vi "acquisition test fixed exposure 4.vi"() -> ()   [LabVIEW 2023]
uses:
  <vilib>/vision/driver/IMAQdx.llb/IMAQdx Attribute Type.ctl
  <vilib>/userDefined/High Color/IMAQdx.ctl
  <vilib>/vision/driver/IMAQdx.llb/IMAQdx Acquisition Mode.ctl
  Program Files/NI/LVAddons/niimaqdx/1/examples/Vision Acquisition/NI-IMAQdx/Stream to Disk/SubVIs/TDMS Write Settings.ctl
  <vilib>/vision/Image Controls.llb/IMAQ Image.ctl
  <vilib>/vision/driver/IMAQdx.llb/IMAQdx Buffer Number Mode.ctl
  <vilib>/DAQmx/read.llb/DAQmx Read (Analog 1D Wfm NChan NSamp).vi
  <extravilib>/ChannelInstances/Tag-bool/Read With Abort.vi
  <vilib>/Utility/High Resolution Relative Seconds.vi
  <extravilib>/ChannelInstances/Tag-bool/Write With Abort.vi
  <vilib>/DAQmx/create/channels.llb/DAQmx Create Channel (AI-Voltage-Basic).vi
  <vilib>/DAQmx/configure/timing.llb/DAQmx Timing (Sample Clock).vi
  Program Files/NI/LVAddons/niimaqdx/1/examples/Vision Acquisition/NI-IMAQdx/Stream to Disk/SubVIs/TDMS File Initialization (Write).vi
  <extravilib>/ChannelInstances/Tag-bool/Instantiate.vi
  <extravilib>/ChannelInstances/Tag-bool/EndpointRead.vi
  <vilib>/vision/EDVR.llb/IMAQ ImageToEDVR.vi
  <vilib>/vision/EDVR.llb/IMAQ ImageToEDVR 1D U8.vi
  <vilib>/vision/EDVR.llb/IMAQ ImageToEDVR 1D I16.vi
  <vilib>/vision/EDVR.llb/IMAQ ImageToEDVR 1D U32.vi
  <vilib>/vision/EDVR.llb/IMAQ ImageToEDVR 1D U16.vi
  <extravilib>/ChannelInstances/Tag-bool/Endpoint.vi
  <vilib>/DAQmx/miscellaneous.llb/DAQmx Fill In Error Info.vi
  <extravilib>/ChannelInstances/Tag-bool.lvlib
  <vilib>/vision/driver/NI_Vision_Acquisition_Software.lvlib
  <resource>/objmgr/imaqdx.rc
panel:
  out "error out":errorcluster
  in  "Image Type":u16(ring) items=["Grayscale (U8)"=0, "Grayscale (I16)"=1, "Grayscale (U16)"=7, "RGB Color (U32)"=4]
  out "Image 2":T1(plugin-control)
  in  "Buffer Images":i32=30
  out "Optimizations":T2
  in  "Images per TDMS":i64=10000
  out "Images Behind 2":u32
  out "Write Speed":dbl(graph) caption="Image File Write Speed"
  out "Images Acquired Per Second":dbl
  out "Images Saved Per Second":dbl
  out "Destination Folder":path
  out "Maximum FrameRate":dbl
  out "Attribute Information":T4
  out "Sensor Readout Time":dbl
  out "Waveform Chart":waveform(dbl)[](graph)
  in  "stop collection":bool
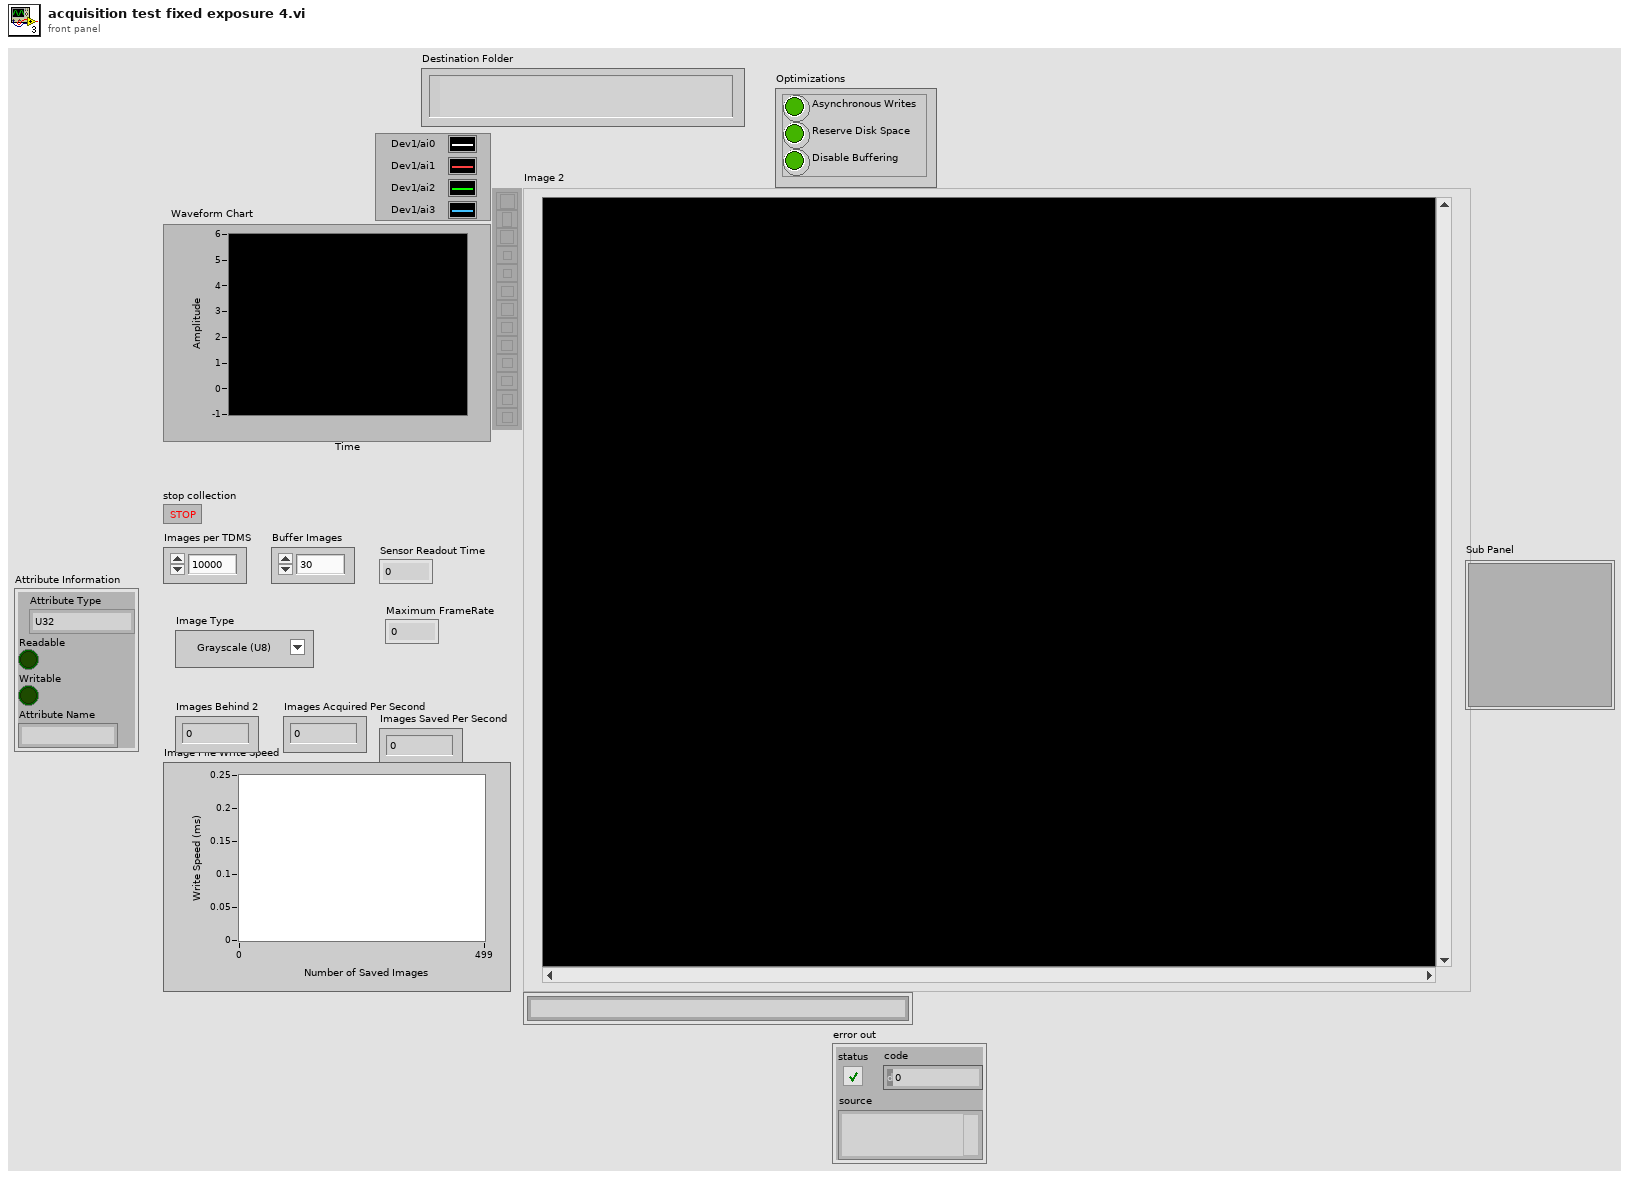
[diagram p1: front panel]
types:
  T1 = typedef "IMAQ Image.ctl" = refnum<image>
  T2 = cluster{"Asynchronous Writes":bool, "Reserve Disk Space":bool, "Disable Buffering":bool}
  T3 = typedef "NI_Vision_Acquisition_Software.lvlib/IMAQdx Attribute Type.ctl" = enum32{"U32", "I64", "DBL", "String", "Enum", "Bool", "Command"}
  T4 = cluster{"Attribute Type":T3, "Readable":bool, "Writable":bool, "Attribute Name":string}
  T5 = typedef "TDMS Write Settings.ctl" = cluster{"Asynchronous":bool, "Disable Buffering if Supported":bool, "Reserved Images":i64, "Fail if Reservation Fails":bool}
  T6 = typedef "NI_Vision_Acquisition_Software.lvlib/IMAQdx Acquisition Mode.ctl" = enum32{"One Shot", "Continuous"}
  T7 = enum16{"Exposure End", "Exposure Center", "Exposure Start", "Start", "NoSync"}
  T8 = typedef "IMAQdx.ctl" = refnum<k21>
  T9 = cluster{"Attribute Type":T3, "Readable":bool, "Writable":bool, "Attribute Name":string}[]
  T10 = typedef "Image Type" = u32
  T11 = cluster{"Image Type":T10, "Async File Format":bool}
  T12 = cluster{"Asynchronous Write":bool, "Reserve Disk Space":bool, "Disable Buffering":bool}
  T13 = typedef "Tag-bool.lvlib/))Channel.ctl" = refnum<queue>
  T14 = typedef "NI_Vision_Acquisition_Software.lvlib/IMAQdx Buffer Number Mode.ctl" = enum32{"Next", "Last", "Buffer Number", "Every", "Last New"}
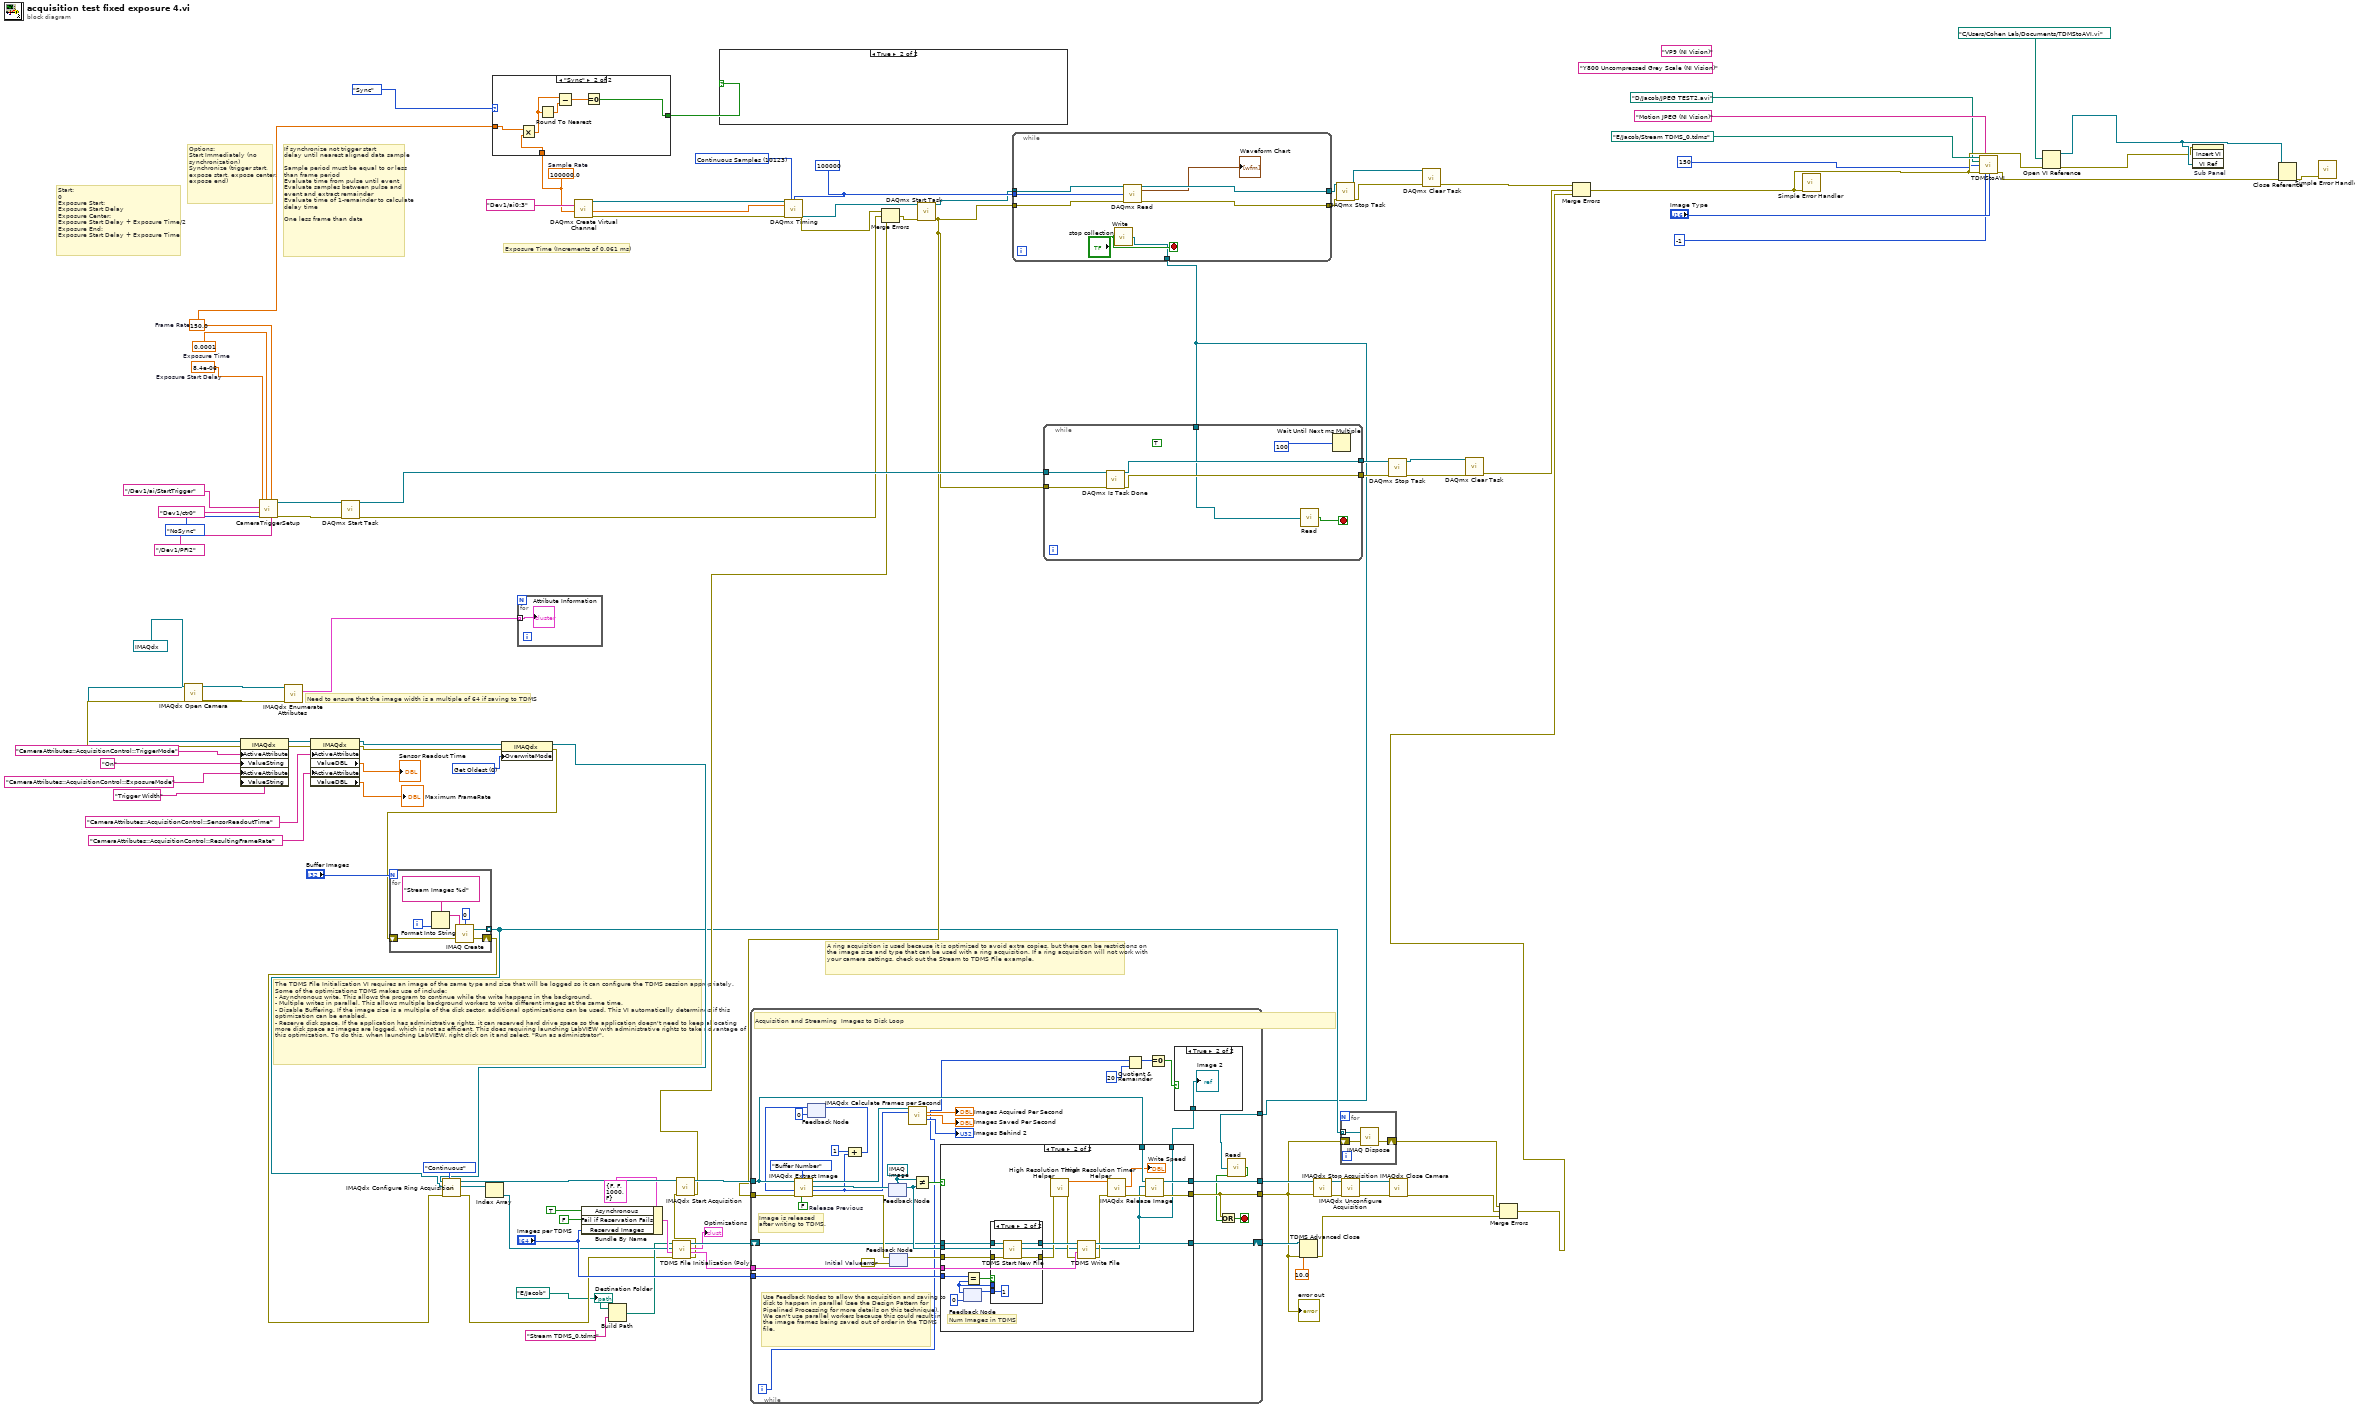
[diagram p0: block diagram]
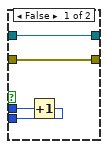
[diagram p4: hidden frame]
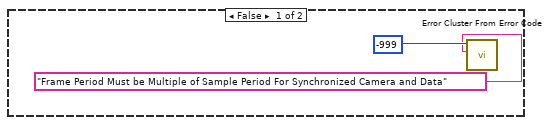
[diagram p5: hidden frame]
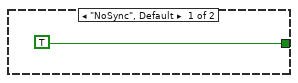
[diagram p6: hidden frame]
diagram:
  w6 = path "E:/Jacob" ("Destination Folder")
  (unwired) "Y800 Uncompressed Grey Scale (NI Vision)" ("Codec")
  (unwired) "VP9 (NI Vision)" ("Codec")
  w33 = u32 0 items=["Get Oldest"=0, "Fail"=2, "Get Newest"=3] ("OverwriteMode")
  w71 = 8.4e-06  # Exposure Start Delay
  w67 = 150.0  # Frame Rate
  w70 = 0.0001  # Exposure Time
  w98 = 10123 items=["Finite Samples"=10178, "Continuous Samples"=10123, "Hardware Timed Single Point"=12522] ("sample mode")
  w99 = 100000 ("number of samples per channel")
  w68 = 100000.0  # Sample Rate
  # "Need to ensure that the image width is a multiple of 64 if saving to TDMS"
  # "The TDMS File Initialization VI requires an image of the same type and size that will be logged so it can configure the TDMS session appropriately. Some of the optimizations TDMS makes use of include:\n- Asynchronous write. This allows the program to continue while the write happens in the background.\n- Multiple writes in parallel. This allows multiple background workers to write different images at the same time.\n- Disable Buffering. If the image size is a multiple of the disk sector, additional optimizations can be used. This VI automatically determines if this optimization can be enabled.\n- Reserve disk space. If the application has administrative rights, it can reserved hard drive space so the application doesn't need to keep allocating more disk space as images are logged, which is not as efficient. This does requiring launching LabVIEW with administrative rights to take advantage of this optimization. To do this, when launching LabVIEW, right click on it and select, \"Run as administrator\"."
  # "A ring acquisition is used because it is optimized to avoid extra copies, but there can be restrictions on the image size and type that can be used with a ring acquisition. If a ring acquisition will not work with your camera settings, check out the Stream to TDMS File example."
  # "Start:\n0\nExposure Start:\nExposure Start Delay\nExposure Center:\nExposure Start Delay + Exposure Time/2\nExposure End:\nExposure Start Delay + Exposure Time"
  # "If synchronize not trigger start\ndelay until nearest aligned data sample\n\nSample period must be equal to or less than frame period\nEvaluate time from pulse until event\nEvaluate samples between pulse and event and extract remainder\nEvaluate time of 1-remainder to calculate delay time\n\nOne less frame than data"
  # "Options:\nStart Immediately (no synchronization)\nSynchronize (trigger start, expose start, expose center, expose end)"
  # "Exposure Time (Increments of 0.061 ms)"
  n1 = call <vilib>:"IMAQdx Open Camera.vi"("Session In"=T8 "cam0") -> ("error out"=w89:errorcluster, "Session Out"=w94:T8)  [unwired: 9 in]
  n2 = call "CameraTriggerSetup.vi"("Camera\nTrigger\nOutput"=tag "/Dev1/PFI2" ("CO.Pulse.Term"), "Frame Rate"=w67, "Sync Type"=T7."NoSync", "Exposure Time"=w70, "Camera\nClock\nCounter"=tag "Dev1/ctr0" ("counter"), "Start Trigger Source"=tag "/Dev1/ai/StartTrigger" ("source"), "Exposure Start Delay"=w71) -> ("error out"=w64:errorcluster, "Refnum out"=w65:refnum<k21>)  [unwired: 3 in]
  n3 = call <vilib>:"IMAQdx Enumerate Attributes.vi"("error in"=w89, "Session In"=w94) -> ("error out"=w93:errorcluster, "Attribute Information Array"=w84:T9, "Session Out"=w92:T8)  [unwired: 7 in]
  n4 = property class="IMAQdx"(reference=w92, error in=w93, "ActiveAttribute"="CameraAttributes::AcquisitionControl::TriggerMode", "ValueString"="On", "ActiveAttribute"="CameraAttributes::AcquisitionControl::ExposureMode", "ValueString"="Trigger Width") -> (reference out=w86:T8, error out=w85:errorcluster)
  n5 = property class="IMAQdx"(reference=w86, error in=w85, "ActiveAttribute"="CameraAttributes::AcquisitionControl::SensorReadoutTime", "ActiveAttribute"="CameraAttributes::AcquisitionControl::ResultingFrameRate") -> (reference out=w32:T8, error out=w31:errorcluster, "ValueDBL"=→"Sensor Readout Time":dbl, "ValueDBL"=→"Maximum FrameRate":dbl)
  n6 = call <vilib>:"DAQmx Start Task.vi"("task/channels in"=w65, "error in"=w64) -> ("task out"=w63:refnum<k21>, "error out"=w58:errorcluster)  [unwired: 12 in]
  n7 = case shown="\"Sync\"" enum16{"NoSync", "Sync"}."Sync" {
    tunnel: [TRUE w104] -> w66
    tunnel: w67 -> [_ w109]
    tunnel: w68 -> [_ w108]
    frame "NoSync", Default {
    }
    frame "Sync" {
      n8 = Multiply(x=w109, y=w108) -> (x*y=w105:dbl)
      n9 = Round To Nearest(number=w105) -> (nearest integer value=w107:dbl)
      n10 = Subtract(x=w105, y=w107) -> (x-y=w106:dbl)
      n11 = Equal To 0?(x=w106) -> (x = 0?=w104:bool)
    }
  }
  n12 = property class="IMAQdx"(reference=w32, error in=w31, "OverwriteMode"=w33) -> (reference out=w25:T8, error out=w29:errorcluster)
  n13 = for {
    N: "Buffer Images" -> [_]
    tunnel: [w115] -> w23 mode=indexing
    shift-right: [w114] -> w24
    shift-left: w29 -> [w116]
    i -> [w113]
    n14 = Format Into String(format string="Stream Images %d" ("Image Name"), w113) -> (resulting string=w112:string)  [unwired: 2 in, 1 out]
    n15 = call "IMAQ Create"("Border Size"=0, "Image Name"=w112, "error in (no error)"=w116) -> ("New Image"=w115:T1, "error out"=w114:errorcluster)  [unwired: 1 in, 1 out]
  }
  n16 = call <vilib>:"IMAQdx Configure Ring Acquisition.vi"("Mode"=IMAQdx_Acquisition_Mode."Continuous" ("Continuous?"), "error in"=w24, "Images"=w23, "Session In"=w25) -> ("error out"=w7:errorcluster, "Images Out"=w36:T1[], "Session Out"=w49:T8)  [unwired: 5 in]
  n17 = Index Array(array=w36) -> (element=w35:T1)  [unwired: 1 in]
  n18 = for {
    tunnel: w84 -> [w117] mode=indexing
    "Attribute Information" <- w117
  }
  n19 = call-poly <vilib>:"DAQmx Create Virtual Channel.vi"("physical channels"=tag "Dev1/ai0:3") -> ("task out"=w102:refnum<k21>, "error out"=w101:errorcluster)  [unwired: 13 in]
  n20 = Bundle By Name(cluster=T5 {"Asynchronous"=FALSE, "Disable Buffering if Supported"=FALSE, "Reserved Images"=1000, "Fail if Reservation Fails"=FALSE} ("Write Settings"), "Asynchronous"=TRUE, "Fail if Reservation Fails"=FALSE, "Reserved Images"="Images per TDMS") -> (w39:T5)
  n21 = Build Path(base path=w6, name or relative path="Stream TDMS_0.tdms") -> (appended path=w20:path)
  n22 = call-poly "TDMS File Initialization (Poly).vi"("error in (no error)"=w7, "Write Settings"=w39, "Image In"=w35, "File Path"=w20) -> ("error out"=w34:errorcluster, "Write Settings Out"=w42:T11, "Optimizations Configured"=→"Optimizations":T12, "TDMS Refnum Out"=w44:refnum<k34>)  [unwired: 4 in]
  n23 = call <vilib>:"IMAQdx Start Acquisition.vi"("error in"=w34, "Session In"=w49) -> ("error out"=w27:errorcluster, "Session Out"=w46:T8)  [unwired: 8 out]
  n24 = case shown="True" w66 {
    frame False {
      n25 = call <vilib>:"Error Cluster From Error Code.vi"("error message (\"\")"="Frame Period Must be Multiple of Sample Period For Synchronized Camera and Data" ("source"), "error code (0)"=-999 ("code")) -> ()  [unwired: 7 in, 1 out]
    }
    frame True {
    }
  }
  n26 = call-poly <vilib>:"DAQmx Timing.vi"("task/channels in"=w102, "sample mode"=w98, "samples per channel"=w99, "rate"=w68, "error in"=w101) -> ("task out"=w62:refnum<k21>, "error out"=w60:errorcluster)  [unwired: 9 in]
  n27 = Merge Errors(w60, w58, w27) -> (w59:errorcluster)
  n28 = call <vilib>:"DAQmx Start Task.vi"("task/channels in"=w62, "error in"=w59) -> ("task out"=w61:refnum<k21>, "error out"=w26:errorcluster)  [unwired: 12 in]
  n29 = while {
    tunnel: [w127] -> w82
    tunnel: [w126] -> w81
    tunnel: w61 -> [w125]
    tunnel: w26 -> [w124]
    tunnel: w99 -> [w123]
    tunnel: [w120] -> w22
    stop <- "stop collection" stop-if-true
    n30 = call <extravilib>:"Write.vi"("element"="stop collection") -> ("channel"=w120:T13)  [unwired: 1 out]
    n31 = call-poly <vilib>:"DAQmx Read.vi"("task/channels in"=w125, "number of samples per channel"=w123, "error in"=w124) -> ("task out"=w127:refnum<k21>, "data"=→"Waveform Chart":waveform(dbl)[], "error out"=w126:errorcluster)  [unwired: 10 in]
  }
  n32 = while {
    tunnel: w26 -> [w161]
    tunnel: w46 -> [w158]
    tunnel: [w159] -> w47
    tunnel: [w147] -> w12
    shift-right: [w160] -> w41
    shift-left: w44 -> [w144]
    tunnel: "Images per TDMS" -> [w143]
    tunnel: w42 -> [w146]
    tunnel: w22 -> [w129]
    i -> [w131]
    stop <- w149 stop-if-true
    w135 = errorcluster {"status"=FALSE, "code"=0, "source"=""}  # Initial Value
    w156 = FALSE  # Release Previous
    w152 = T1 refnum ("Image Out")
    # "Use Feedback Nodes to allow the acquisition and saving to disk to happen in parallel (see the Design Pattern for Pipelined Processing for more details on this technique). We can't use parallel workers because this could result in the image frames being saved out of order in the TDMS file."
    # "Image is released after writing to TDMS."
    # "Acquisition and Streaming  Images to Disk Loop"
    n33 = feedback #1(u32 0) -> (w137:u32)
    n34 = call <vilib>:"IMAQdx Extract Image.vi"("Release Previous (true)"=w156, "Buffer Number Mode (Next)"=IMAQdx_Buffer_Number_Mode."Buffer Number" ("Buffer Number Mode"), "error in"=w161, "Buffer Number In"=w137, "Session In"=w158) -> ("error out"=w145:errorcluster, "Buffer Number Out"=w139:u32, "Image Out"=w154:T1, "Session Out"=w155:T8)  [unwired: 3 in]
    n35 = Compound Arithmetic op=ADD(u32 1 ("value"), w139) -> (w140:u32)
    n36 = feedback-in #1(w140) -> ()
    n37 = feedback-in #2(w154) -> ()
    n38 = feedback #2(w152) -> (w150:T1)
    n39 = feedback-in #3(w145) -> ()
    n40 = feedback #3(w135) -> (w153:errorcluster)
    n41 = call <vilib>:"IMAQdx Calculate Frames per Second.vi"("Session In"=w155, "Buffer Number"=w139) -> ("Acquired Frames per Second"=→"Images Acquired Per Second":dbl, "Processed Frames per Second"=→"Images Saved Per Second":dbl, "Images Behind"=→"Images Behind 2":i32)  [unwired: 7 in, 4 out]
    n42 = Not Equal?(x=w152, y=w150) -> (x != y?=w151:bool)
    n43 = case shown="True" w151 {
      tunnel: w144 -> [w164 w180]
      tunnel: w150 -> [w163 w167]
      tunnel: w153 -> [w165 w178]
      tunnel: [w164 w183] -> w160
      tunnel: [w166 w186] -> w159
      tunnel: w158 -> [w166 w185]
      tunnel: [w165 w184] -> w147
      tunnel: w146 -> [_ w182]
      tunnel: w143 -> [_ w176]
      tunnel: [w163 w167] -> w130
      frame False {
        # "First iteration doesn't have valid image for this pipelined stage."
      }
      frame True {
        # "Num Images in TDMS"
        n44 = feedback #4(i64 0) -> (w175:i64)
        n45 = Equal?(x=w176, y=w175) -> (x = y?=w177:bool)
        n46 = case shown="True" w177 {
          tunnel: [w190 i64 1] -> w174
          tunnel: w180 -> [w189 w194]
          tunnel: [w189 w193] -> w179
          tunnel: w178 -> [w188 w191]
          tunnel: [w188 w192] -> w173
          tunnel: w175 -> [w187 _]
          frame False {
            n47 = Increment(x=w187) -> (x+1=w190:i64)
          }
          frame True {
            n48 = call "TDMS Start New File.vi"("error in"=w191, "Previous TDMS Refnum In"=w194) -> ("error out"=w192:errorcluster, "New TDMS Refnum Out"=w193:refnum<k34>)  [unwired: 8 in]
          }
        }
        n49 = feedback-in #4(w174) -> ()
        n50 = call "High Resolution Timer Helper.vi"("error in (no error)"=w173) -> ("error out"=w172:errorcluster, "Current Time"=w170:dbl)  [unwired: 8 in, 1 out]
        n51 = call "TDMS Write File.vi"("error in"=w172, "Write Settings"=w182, "Image"=w167, "TDMS Ref In"=w179) -> ("error out"=w171:errorcluster, "TDMS Ref Out"=w183:refnum<k34>)  [unwired: 6 in]
        n52 = call "High Resolution Timer Helper.vi"("error in (no error)"=w171, "Previous Time"=w170) -> ("error out"=w169:errorcluster, "Time Difference (ms)"=→"Write Speed":dbl)  [unwired: 7 in, 1 out]
        n53 = call <vilib>:"IMAQdx Release Image.vi"("error in"=w169, "Image"=w167, "Session In"=w185) -> ("error out"=w184:errorcluster, "Session Out"=w186:T8)  [unwired: 7 in]
      }
    }
    n54 = Quotient & Remainder(x=w131, y=20) -> (x-y*floor(x/y)=w134:i32)  [unwired: 1 out]
    n55 = Equal To 0?(x=w134) -> (x = 0?=w133:bool)
    n56 = case shown="True" w133 {
      tunnel: w130 -> [_ w162]
      frame False {
      }
      frame True {
        "Image 2" <- w162
      }
    }
    n57 = call <extravilib>:"Read.vi"("channel"=w129) -> ("element"=w128:bool)  [unwired: 1 in, 1 out]
    n58 = Or(x=w147, y=w128) -> (x .or. y?=w149:bool)
  }
  "error out" <- w12
  n59 = while {
    tunnel: w22 -> [w196]
    tunnel: w63 -> [w201]
    tunnel: w26 -> [w200]
    tunnel: [w199] -> w78
    tunnel: [w198] -> w77
    stop <- w202 stop-if-true
    (unwired) TRUE ("auto start")
    n60 = call <vilib>:"DAQmx Is Task Done.vi"("task/channels in"=w201, "error in"=w200) -> ("task out"=w199:refnum<k21>, "error out"=w198:errorcluster)  [unwired: 11 in, 1 out]
    n61 = call <extravilib>:"Read.vi"("channel"=w196) -> ("element"=w202:bool)  [unwired: 1 in, 1 out]
    n62 = Wait Until Next ms Multiple(millisecond multiple=u32 100) -> ()  [unwired: 1 out]
  }
  n63 = TDMS Advanced Close(6:10.0 ("timeout (10 s)"), 8:w12, 11:w41) -> (0:w15:errorcluster)  [unwired: 1 in, 1 out]
  n64 = call <vilib>:"IMAQdx Stop Acquisition.vi"("error in"=w12, "Session In"=w47) -> ("error out"=w50:errorcluster, "Session Out"=w51:T8)  [unwired: 8 out]
  n65 = call <vilib>:"DAQmx Stop Task.vi"("task/channels in"=w82, "error in"=w81) -> ("task out"=w80:refnum<k21>, "error out"=w57:errorcluster)  [unwired: 12 in]
  n66 = for {
    shift-right: [w204] -> w13
    shift-left: w12 -> [w205]
    tunnel: w23 -> [w203] mode=indexing
    n67 = call "IMAQ Dispose"("Image"=w203, "error in (no error)"=w205) -> ("error out"=w204:errorcluster)  [unwired: 4 in]
  }
  n68 = call <vilib>:"IMAQdx Unconfigure Acquisition.vi"("error in"=w50, "Session In"=w51) -> ("error out"=w53:errorcluster, "Session Out"=w52:T8)  [unwired: 8 out]
  n69 = call <vilib>:"DAQmx Stop Task.vi"("task/channels in"=w78, "error in"=w77) -> ("task out"=w83:refnum<k21>, "error out"=w56:errorcluster)  [unwired: 12 in]
  n70 = call <vilib>:"IMAQdx Close Camera.vi"("error in"=w53, "Session In"=w52) -> ("error out"=w14:errorcluster)  [unwired: 9 out]
  n71 = call <vilib>:"DAQmx Clear Task.vi"("task in"=w80, "error in"=w57) -> ("error out"=w55:errorcluster)  [unwired: 13 in]
  n72 = call <vilib>:"DAQmx Clear Task.vi"("task in"=w83, "error in"=w56) -> ("error out"=w54:errorcluster)  [unwired: 13 in]
  n73 = Merge Errors(w13, w14, w15) -> (w5:errorcluster)
  n74 = Merge Errors(w55, w54, w5) -> (w10:errorcluster)
  n75 = call <vilib>:"Simple Error Handler.vi"("error in (no error)"=w10) -> ()  [unwired: 4 in, 5 out]
  n76 = call "TDMStoAVI.vi"("TDMS Path"=path "E:/Jacob/Stream TDMS_0.tdms" ("AVI Path"), "Codec"="Motion JPEG (NI Vision)", "AVI Out Path"=path "D:/Jacob/JPEG TEST2.avi" ("AVI Path"), "Frames Per Second"=u32 150, "error in (no error)"=w10, "Quality"=-1, "Image Type"="Image Type") -> ("error out"=w9:errorcluster)  [unwired: 8 in]
  n77 = Open VI Reference(vi path=path "C:/Users/Cohen Lab/Documents/TDMStoAVI.vi", error in (no error)=w10) -> (vi reference=w17:refnum<vi>, error out=w11:errorcluster)  [unwired: 4 in]
  n78 = invoke on="Sub Panel" class="SubPnl" method="Insert VI"(error in=w11, "VI Ref"=w17) -> ()  [unwired: 2 in, 4 out]
  n79 = Close Reference(reference=w17, error in (no error)=w9) -> (error out=w8:errorcluster)
  n80 = call <vilib>:"Simple Error Handler.vi"("error in (no error)"=w8) -> ()  [unwired: 4 in, 5 out]
  "Destination Folder" <- w6
